vi "Start.vi"(8 "error in (no error)":errorcluster, 11 "DiscoveryService in":refnum<class "DiscoveryService.lvclass">) -> (0 "error out":errorcluster, 3 "DiscoveryService out":refnum<class "DiscoveryService.lvclass">)   [LabVIEW 2020, in "Vecto.lvlib" / "DiscoveryService.lvclass"]
uses:
  DiscoveryService.lvclass
  DiscoveryService.lvclass/DiscoveryService.ctl
  <vilib>/Utility/tcp.llb/UDP Multicast Read-Write Open.vi
  Discovery Loop Async.vi
  Node Config/Node Config.lvclass
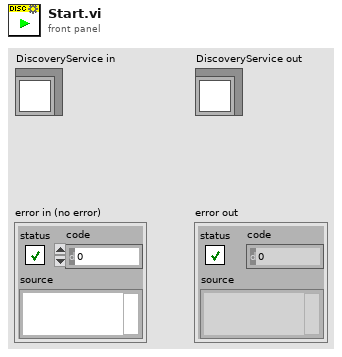
[diagram p1: front panel]
types:
  T1 = typedef "VectoConfig.lvlib/Node Config.lvclass/Discovery Info.ctl" = cluster{"Address":string, "Port":u16, "Interval S":dbl, "Bind Address":string}
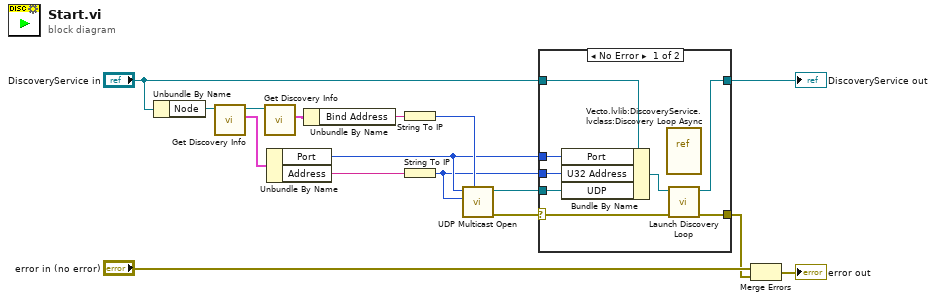
[diagram p0: block diagram]
diagram:
  n1 = Unbundle By Name("DiscoveryService in") -> ("Node"=w16:refnum<class "Node Config.lvclass">)
  n2 = call "Get Discovery Info.vi"("Node in"=w16) -> ("Discovery Info"=w15:T1, "Node out"=w13:refnum<class "Node Config.lvclass">)  [unwired: 8 in, 1 out]
  n3 = call "Get Discovery Info.vi"("Node in"=w13) -> ("Discovery Info"=w2:T1)  [unwired: 8 in, 2 out]
  n4 = Unbundle By Name(w15) -> ("Port"=w10:u16, "Address"=w14:string)
  n5 = Unbundle By Name(w2) -> ("Bind Address"=w1:string)
  n6 = String To IP(1:w1) -> (0:w12:u32)
  n7 = String To IP(1:w14) -> (0:w9:u32)
  n8 = call-poly <vilib>:"UDP Multicast Open.vi"("net address"=w12, "multicast addr"=w9, "port"=w10) -> ("error out"=w4:errorcluster, "connection ID"=w8:refnum<k16>)  [unwired: 6 in, 1 out]
  n9 = case shown="No Error" w4 {
    selector: w4 -> [w18 w25]
    tunnel: "DiscoveryService in" -> [w24 w26]
    tunnel: w10 -> [w23 _]
    tunnel: w9 -> [w22 _]
    tunnel: w8 -> [w21 _]
    tunnel: [w19 w26] -> w7
    tunnel: [w17 w25] -> w3
    frame No Error {
      n10 = Bundle By Name(cluster=w24, "Port"=w23, "U32 Address"=w22, "UDP"=w21) -> (w20:refnum<class "DiscoveryService.lvclass">)
      n11 = vi-ref "Vecto.lvlib:DiscoveryService.lvclass:Discovery Loop Async.vi"() -> ()  [unwired: 1 out]
      n12 = call "Launch Discovery Loop.vi"("error in (no error)"=w18, "DiscoveryService in"=w20) -> ("error out"=w17:errorcluster, "DiscoveryService out"=w19:refnum<class "DiscoveryService.lvclass">)  [unwired: 8 in]
    }
    frame Error {
    }
  }
  "DiscoveryService out" <- w7
  n13 = Merge Errors("error in (no error)", w3) -> (→"error out":errorcluster)
